vi "Close Log File camera.vi"(8 "error in (no error)":errorcluster, 11 "AVI Refnum in":T1) -> (0 "error out":errorcluster)   [LabVIEW 2017]
uses:
  <vilib>/vision/Avi.llb/IMAQ AVI2 Refnum.ctl
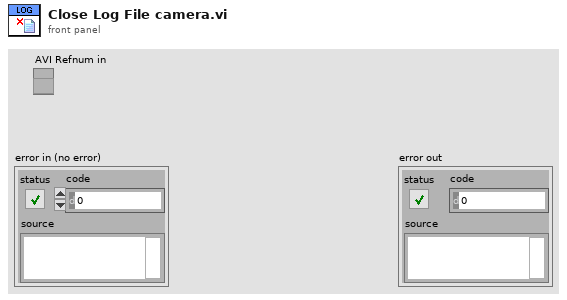
[diagram p1: front panel]
types:
  T1 = typedef "IMAQ AVI2 Refnum.ctl" = refnum<k20>
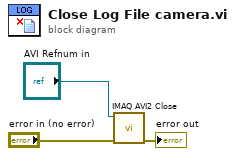
[diagram p0: block diagram]
diagram:
  n1 = call "IMAQ AVI2 Close"("error in (no error)"="error in (no error)", "AVI Refnum"="AVI Refnum in") -> ("error out"=→"error out":errorcluster)  [unwired: 9 in]
